vi "Default Read Before Fulfill.vi"(8 "error in (no error)":errorcluster) -> (0 "error out":errorcluster)   [LabVIEW 2017, in "Unit Tests.lvlib"]
uses:
  Unit Tests.lvlib
  c664d439-2256-4a9f-a739-dc12c290693a.vi
  aabc8cba-9084-4be5-a205-3220d6b46a01.vi
  b9a04ffe-19ac-44ac-a98a-535b1aadafcc.vi
  Promise Future/Promise/Promise.lvclass
  E:/Promise/Promise Future/Future/Future.lvclass
  Promise Future/Promise/Read Future.vi
  Promise Future/Future/Read Value (private).vi
  Promise Future/Future/Fulfull (Value).vi
  Promise Future/Future/Future.lvclass
  <vilib>/addons/_JKI Toolkits/Caraya/classes/Test/Test.lvclass
  <vilib>/addons/_JKI Toolkits/Caraya/classes/Assert/Assert.lvclass
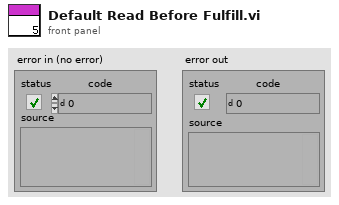
[diagram p1: front panel]
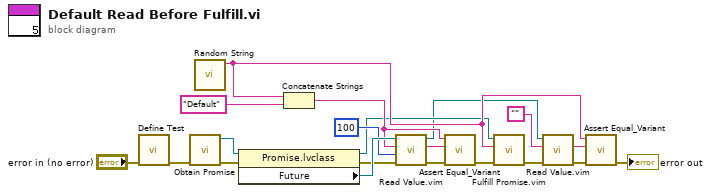
[diagram p0: block diagram]
diagram:
  n1 = call <vilib>:"Define Test.vi"("error in (no error)"="error in (no error)") -> ("error out"=w16:errorcluster)  [unwired: 10 in]
  n2 = call "Obtain Promise.vi"("error in (no error)"=w16) -> ("error out"=w20:errorcluster, "Promise out"=w15:refnum<class "Promise.lvclass">)  [unwired: 8 in, 1 out]
  n3 = call "Random String.vi"() -> ("string"=w11:string)  [unwired: 11 in]
  n4 = property class="Promise.lvclass"(reference=w15, error in=w20) -> (reference out=w2:refnum<class "Promise.lvclass">, error out=w18:errorcluster, "Future"=w19:refnum<class "Future.lvclass">)
  n5 = Concatenate Strings(w11, "Default" ("String")) -> (w5:string)
  n6 = call "Read Value.vim"("error in (no error)"=w18, "timeout in ms (-1)"=u32 100 ("milliseconds to wait"), "Default Value"=w5, "Future in"=w19) -> ("error out"=w8:errorcluster, "Value"=w6:string, "Future out"=w1:refnum<class "Future.lvclass">)  [unwired: 4 in, 1 out]
  n7 = call <vilib>:"Assert Equal_Variant.vi"("error in (no error)"=w8, "Y"=w6, "X"=w5) -> ("error out"=w7:errorcluster)  [unwired: 8 in]
  n8 = call "Fulfill Promise.vim"("error in (no error)"=w7, "Value"=w11, "Promise in"=w2) -> ("error out"=w10:errorcluster)  [unwired: 7 in, 1 out]
  n9 = call "Read Value.vim"("error in (no error)"=w10, "Default Value"="", "Future in"=w1) -> ("error out"=w9:errorcluster, "Value"=w3:string)  [unwired: 5 in, 2 out]
  n10 = call <vilib>:"Assert Equal_Variant.vi"("error in (no error)"=w9, "Y"=w3, "X"=w11) -> ("error out"=→"error out":errorcluster)  [unwired: 8 in]
